vi "Heater_Setpoint_Panel.vi"() -> ()   [LabVIEW 2013]
uses:
  Heater_Setpoint.ctl
  ADAM Controls/Channel_names.ctl
  ADAM Controls/Update_scan_value.ctl
  ADAM Controls/Channel_State.ctl
panel:
  in  "Mode":u16(ring) items=["Only Show Setpoints Above Zero", "Show all Setpoints"]
  in  "Setpoints Out":T1[](array[typedef])
  out "Messages":string
  in  "OK":bool
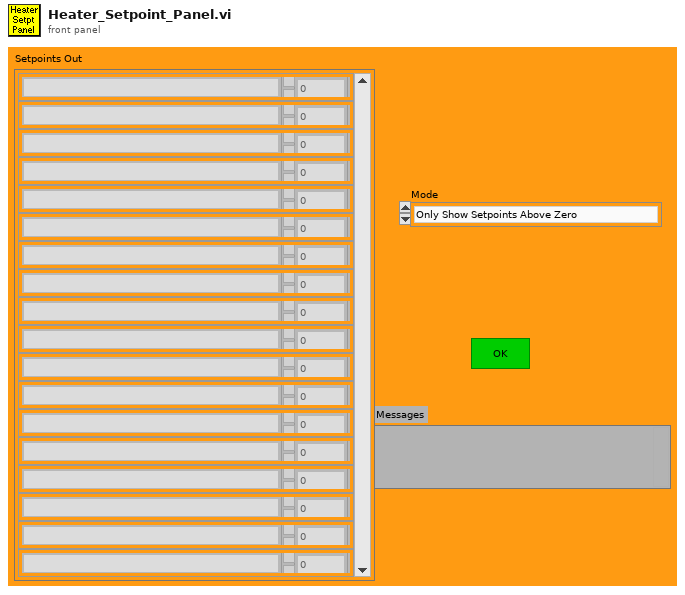
[diagram p1: front panel]
types:
  T1 = typedef "Heater_Setpoint.ctl" = cluster{"Ch Name":string, "Setpoint":dbl}
  T2 = typedef "Channel_names.ctl" = enum16{"Active Only", "Active + Off", "All Channels"}
  T3 = typedef "Update_scan_value.ctl" = cluster{"Channel Name":string, "New Value":dbl}
  T4 = typedef "Channel_State.ctl" = enum16{"On", "Off", "Always On", "Always Off"}
  T5 = typedef "Ch_description_ADAM.ctl" = cluster{"Ch Name":string, "Type":T6, "Function":T7, "Ch State":T4, "Calibration type":T8, "A":dbl, "B":dbl, "C":dbl, "D":dbl, "Comments":string, "Address":T9, "String":string, "Duty":u16}
  T6 = typedef "Module_type_ADAM.ctl" = string
  T7 = typedef "Function_ADAM.ctl" = enum16{"Analogue Input", "Digital Input", "Event counter", "Event rate", "Analogue Output", "Digital Output", "Relay Output"}
  T8 = typedef "Calib_type_ADAM.ctl" = enum16{"Raw", "Bx + A", "Cx^2 + Bx + A", "Dx^3 + Cx^2 + Bx + A", "In Band", "Hi-Tec Q", "Hi-Tec M_dot", "Text"}
  T9 = typedef "Address.ctl" = cluster{"Main":i32, "Ch.":i32, "Sub":i32, "Port Name":string}
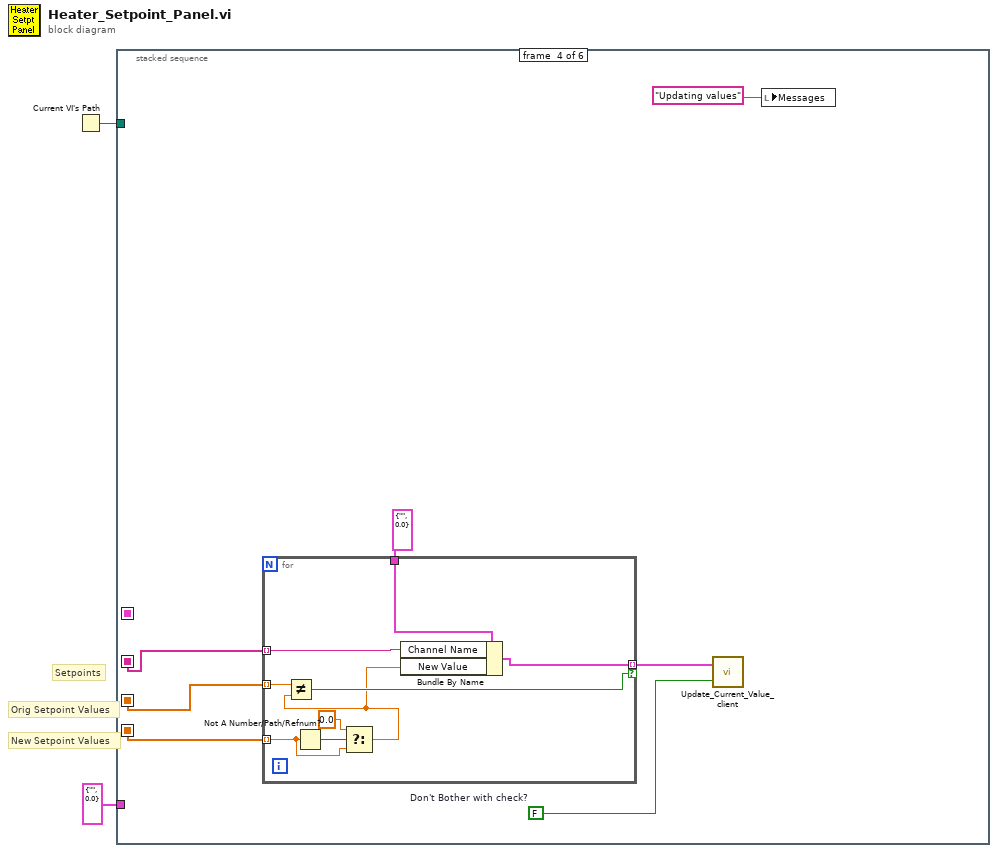
[diagram p0: block diagram]
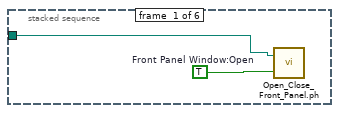
[diagram p2: hidden frame]
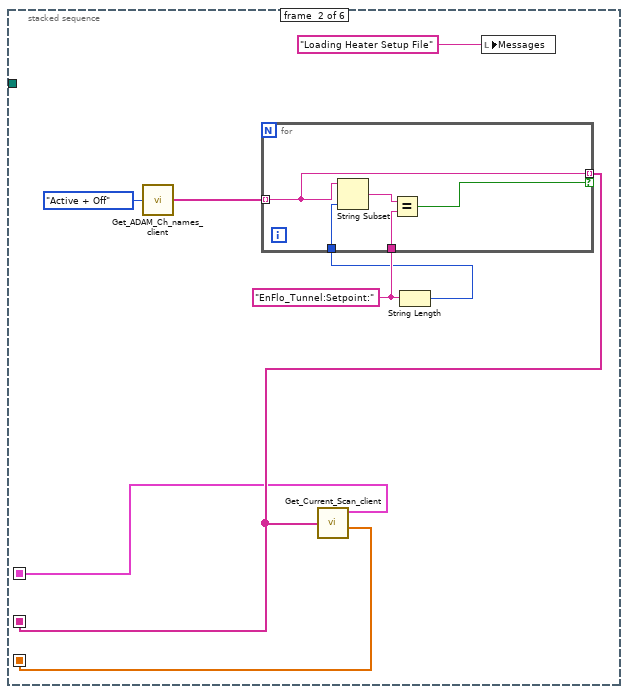
[diagram p3: hidden frame]
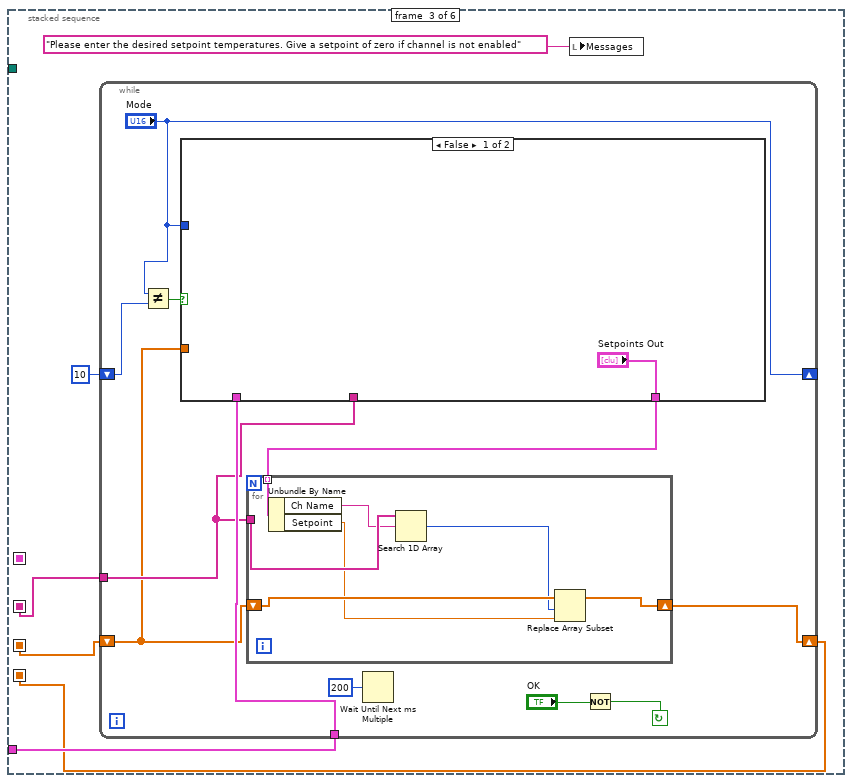
[diagram p4: hidden frame]
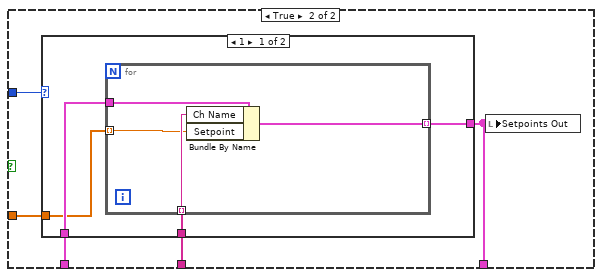
[diagram p5: hidden frame]
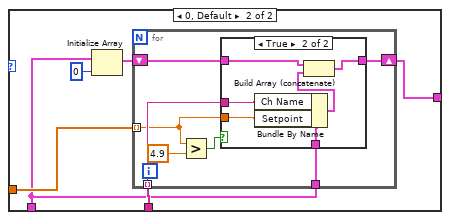
[diagram p6: hidden frame]
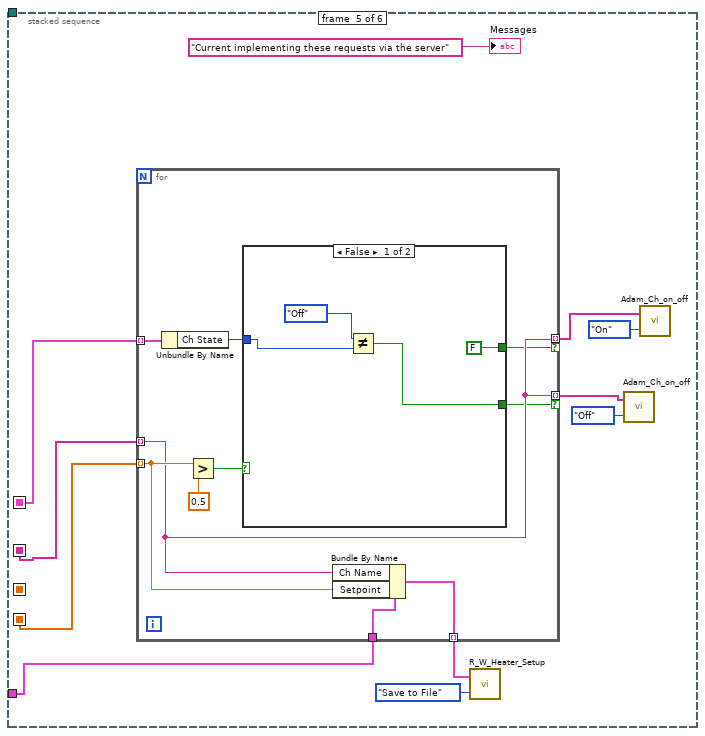
[diagram p8: hidden frame]
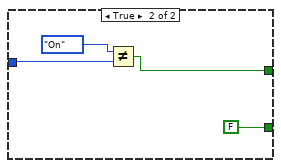
[diagram p9: hidden frame]
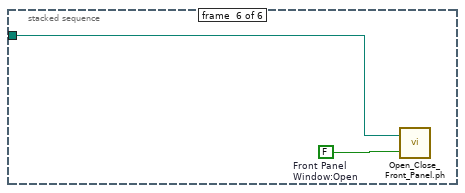
[diagram p10: hidden frame]
diagram:
  # "New Setpoint Values"
  # "Orig Setpoint Values"
  # "Setpoints"
  n1 = Current VI's Path() -> (path=w2:path)
  n2 = stacked-sequence {
    seq-local: [_ w7 _ _ _ _] -> [_ _ w20 w77 _ _]
    seq-local: [_ w6 _ _ _ _] -> [_ _ w22 w80 w99 _]
    seq-local: [_ _ w18 _ _ _] -> [_ _ _ w79 w98 _]
    seq-local: [_ w5 _ _ _ _] -> [_ _ _ _ w92 _]
    tunnel: w2 -> [w4 _ _ _ _ w121]
    tunnel: T1 {"Ch Name"="", "Setpoint"=0.0} ("Cluster") -> [_ _ w21 _ w97 _]
    frame #0 {
      w3 = TRUE  # Front Panel Window:Open
      n3 = call "Open_Close_Front_Panel.ph.vi"("Front Panel Window:Open"=w3, "VI path"=w4) -> ()  [unwired: 2 out]
    }
    frame #1 {
      w11 = "EnFlo_Tunnel:Setpoint:"
      n4 = call "Get_ADAM_Ch_names_client.vi"("Channel names set"=Channel_names."Active + Off") -> ("Ch names"=w8:string[])
      n5 = String Length(string=w11) -> (length=w10:i32)
      n6 = for {
        tunnel: w8 -> [w14] mode=indexing
        tunnel: w10 -> [w17]
        tunnel: w11 -> [w16]
        tunnel: [w14] -> w6 mode=indexing if=w13
        n7 = String Subset(string=w14, length (rest)=w17) -> (substring=w15:string)  [unwired: 1 out]
        n8 = Equal?(x=w15, y=w16) -> (x = y?=w13:bool)
      }
      n9 = call "Get_Current_Scan_client.vi"("ADAM Ch Names"=w6) -> ("Ch Description Array"=w5:T5[], "Numerical Values"=w7:dbl[])  [unwired: 2 out]
      n10 = local write "Messages"("Loading Heater Setup File" ("Messages")) -> ()
    }
    frame #2 {
      n11 = while {
        tunnel: w22 -> [w26]
        tunnel: w21 -> [w27]
        shift-right: [w31] -> w18
        shift-left: w20 -> [w25]
        shift-right: ["Mode"] -> _
        shift-left: u16 10 ("Mode") -> [w30]
        stop <- w33 continue-if-true
        n12 = Not Equal?(x="Mode", y=w30) -> (x != y?=w29:bool)
        n13 = case shown="False" w29 {
          tunnel: "Mode" -> [_ w40]
          tunnel: w27 -> [_ w39]
          tunnel: w26 -> [_ w38]
          tunnel: w25 -> [_ w37]
          tunnel: ["Setpoints Out" w36] -> w24
          frame False {
          }
          frame True {
            n14 = case shown="1" w40 {
              tunnel: w39 -> [w44 w51]
              tunnel: w38 -> [w43 w53]
              tunnel: w37 -> [w42 w54]
              tunnel: [w41 w52] -> w36
              frame 1 {
                n15 = for {
                  tunnel: w44 -> [w48]
                  tunnel: w43 -> [w47] mode=indexing
                  tunnel: w42 -> [w46] mode=indexing
                  tunnel: [w45] -> w41 mode=indexing
                  n16 = Bundle By Name(cluster=w48, "Ch Name"=w47, "Setpoint"=w46) -> (w45:T1)
                }
              }
              frame 0, Default {
                n17 = Initialize Array(w51, 0 ("dimension size")) -> (w49:T1[])
                n18 = for {
                  tunnel: w53 -> [w61] mode=indexing
                  tunnel: w54 -> [w60] mode=indexing
                  tunnel: w51 -> [w57]
                  shift-right: [w56] -> w52
                  shift-left: w49 -> [w55]
                  n19 = Greater?(x=w60, y=4.9) -> (0:w58:bool)
                  n20 = case shown="True" w58 {
                    tunnel: w61 -> [_ w68]
                    tunnel: w60 -> [_ w67]
                    tunnel: w57 -> [_ w66]
                    tunnel: [w62 w64] -> w56
                    tunnel: w55 -> [w62 w63]
                    frame False {
                    }
                    frame True {
                      n21 = Bundle By Name(cluster=w66, "Ch Name"=w68, "Setpoint"=w67) -> (w65:T1)
                      n22 = Build Array (concatenate)(w63, w65) -> (w64:T1[])
                    }
                  }
                }
              }
            }
            n23 = local write "Setpoints Out"(w36) -> ()
          }
        }
        n24 = for {
          tunnel: w26 -> [w75]
          shift-right: [w72] -> w31
          shift-left: w25 -> [w73]
          tunnel: w24 -> [w69] mode=indexing
          n25 = Unbundle By Name(w69) -> ("Ch Name"=w74:string, "Setpoint"=w70:dbl)
          n26 = Search 1D Array(1D array=w75, element=w74) -> (index of element=w71:i32)  [unwired: 1 out]
          n27 = Replace Array Subset(array=w73, new element=w70, index=w71) -> (w72:dbl[])
        }
        n28 = Wait Until Next ms Multiple(millisecond multiple=u32 200) -> ()  [unwired: 1 out]
        n29 = Not(x="OK") -> (.not. x?=w33:bool)
      }
      n30 = local write "Messages"("Please enter the desired setpoint temperatures. Give a setpoint of zero if channel is not enabled" ("Messages")) -> ()
    }
    frame #3 {
      w78 = FALSE  # Don't Bother with check?
      n31 = for {
        tunnel: T3 {"Channel Name"="", "New Value"=0.0} ("Update Scan Value Cluster") -> [w91]
        tunnel: w80 -> [w90] mode=indexing
        tunnel: w79 -> [w85] mode=indexing
        tunnel: w77 -> [w89] mode=indexing
        tunnel: [w88] -> w76 mode=indexing if=w87
        n32 = Not A Number/Path/Refnum?(number/path/refnum=w85) -> (NaN/Path/Refnum?=w86:bool)
        n33 = Select(t=0.0, s=w86, f=w85) -> (s? t:f=w83:dbl)
        n34 = Not Equal?(x=w89, y=w83) -> (x != y?=w87:bool)
        n35 = Bundle By Name(cluster=w91, "Channel Name"=w90, "New Value"=w83) -> (w88:T3)
      }
      n36 = call "Update_Current_Value_client.vi"("Don't Bother with check?"=w78, "Update array in"=w76) -> ()
      n37 = local write "Messages"("Updating values" ("Messages")) -> ()
    }
    frame #4 {
      n38 = for {
        tunnel: w99 -> [w108] mode=indexing
        tunnel: w98 -> [w110] mode=indexing
        tunnel: w97 -> [w112]
        tunnel: [w111] -> w96 mode=indexing
        tunnel: [w108] -> w94 mode=indexing if=w107
        tunnel: [w108] -> w93 mode=indexing if=w106
        tunnel: w92 -> [w105] mode=indexing
        n39 = Unbundle By Name(w105) -> ("Ch State"=w103:T4)
        n40 = Greater?(x=w110, y=0.5) -> (0:w104:bool)
        n41 = case shown="False" w104 {
          tunnel: [FALSE w118] -> w107
          tunnel: [w113 FALSE] -> w106
          tunnel: w103 -> [w115 w119]
          frame False {
            n42 = Not Equal?(x=Channel_State."Off" ("Ch State"), y=w115) -> (x != y?=w113:bool)
          }
          frame True {
            n43 = Not Equal?(x=Channel_State."On" ("Ch State"), y=w119) -> (x != y?=w118:bool)
          }
        }
        n44 = Bundle By Name(cluster=w112, "Ch Name"=w108, "Setpoint"=w110) -> (w111:T1)
      }
      n45 = call "R_W_Heater_Setup.vi"("Mode"=enum16{"Load from File", "Save to File"}."Save to File", "Setpoints In"=w96) -> ()  [unwired: 2 out]
      n46 = call "Adam_Ch_on_off.vi"("Ch State"=Channel_State."Off", "ADAM Ch Names"=w93) -> ()  [unwired: 1 out]
      n47 = call "Adam_Ch_on_off.vi"("Ch State"=Channel_State."On", "ADAM Ch Names"=w94) -> ()  [unwired: 1 out]
      "Messages" <- "Current implementing these requests via the server" ("Messages")
    }
    frame #5 {
      w122 = FALSE  # Front Panel Window:Open
      n48 = call "Open_Close_Front_Panel.ph.vi"("Front Panel Window:Open"=w122, "VI path"=w121) -> ()  [unwired: 2 out]
    }
  }
